vi "Difference Quotient, Multi-point.vi"(2 "# of points per slope":i16=2, 3 "X":dbl[](array[numeric]), 4 "Y":dbl[](array[numeric])) -> (1 "dY/dX":dbl[](array[numeric]))   [LabVIEW 2010]
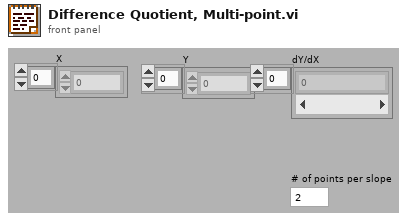
[diagram p1: front panel]
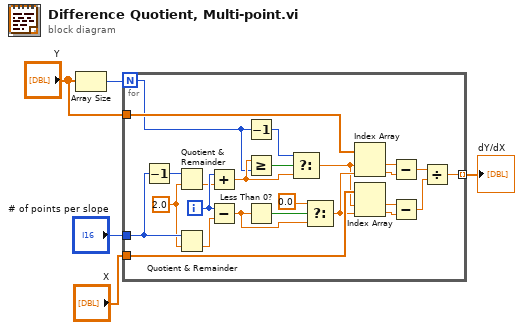
[diagram p0: block diagram]
diagram:
  n1 = Array Size(array="Y") -> (size(s)=w1:i32)
  n2 = for {
    N: w1 -> [w9]
    tunnel: "Y" -> [w29]
    tunnel: "X" -> [w27]
    tunnel: [w25] -> w4 mode=indexing
    tunnel: "# of points per slope" -> [w24]
    i -> [w21]
    w22 = 2.0 ("y")
    n3 = Decrement(x=w24) -> (x-1=w23:i16)
    n4 = Quotient & Remainder(x=w23, y=w22) -> (floor(x/y)=w15:dbl)  [unwired: 1 out]
    n5 = Quotient & Remainder(x=w24, y=w22) -> (floor(x/y)=w16:dbl)  [unwired: 1 out]
    n6 = Add(x=w21, y=w15) -> (x+y=w10:dbl)
    n7 = Subtract(x=w21, y=w16) -> (x-y=w12:dbl)
    n8 = Decrement(x=w9) -> (x-1=w8:i32)
    n9 = Greater Or Equal?(x=w10, y=w9) -> (x >= y?=w11:bool)
    n10 = Less Than 0?(x=w12) -> (x < 0?=w14:bool)
    n11 = Select(t=w8, s=w11, f=w10) -> (s? t:f=w6:dbl)
    n12 = Select(t=0.0 ("x-y"), s=w14, f=w12) -> (s? t:f=w7:dbl)
    n13 = Index Array(array=w29, index #1=w6, index #2=w7) -> (element #1=w20:dbl, element #2=w19:dbl)
    n14 = Index Array(array=w27, index #1=w6, index #2=w7) -> (element #1=w18:dbl, element #2=w17:dbl)
    n15 = Subtract(x=w20, y=w19) -> (x-y=w28:dbl)
    n16 = Subtract(x=w18, y=w17) -> (x-y=w26:dbl)
    n17 = Divide(x=w28, y=w26) -> (x/y=w25:dbl)
  }
  "dY/dX" <- w4
